vi "INIT_HP_2.vi"(4 "Averaging Number (8:256)":u32(ring) items=["1", "2", "4", "8", "16", "32", "64", "128", "256"], 6 "Integration Time":u32(ring)=2 items=["Short", "Medium", "Long"], 7 "Osc_Level [V]":dbl=0.02, 8 "Sweep Mode (0:Repeat)":u32(ring)=2 items=["Repeat", "Single", "Manual Point Mode"], 9 "Set":u32(ring)=7 caption="Selection A-B:" items=["| Z | -Ttheta ", "R - X", "Ls-Rs", "Ls-Q", "Cs-Rs", "Cs-Q", "Cs-D", "|Y|-Theta", "G-B", "Lp-G", "Lp-Q", "Cp-G", "Cp-Q", "Cp-D", "|Z|-Ls", "|Z|-Cs", "|Z|-Lp", "|Z|-Cp", "Lp-Rp", "Cp-Rp"], 10 "Reset Device (T:Reset Device)":bool, 11 "Type":u32(ring) caption="Measurement type" items=["Impedance ", "Gain - Phase", "Impedance With Probe"]) -> (0 "error out":errorcluster, 3 "VISA Refnum out":refnum<visa-resource-name>)   [LabVIEW 2017]
uses:
  ES2M_Auxetico/Lanzi_Romano/VI/Agilent 4194/Agilent 4194.lvlib
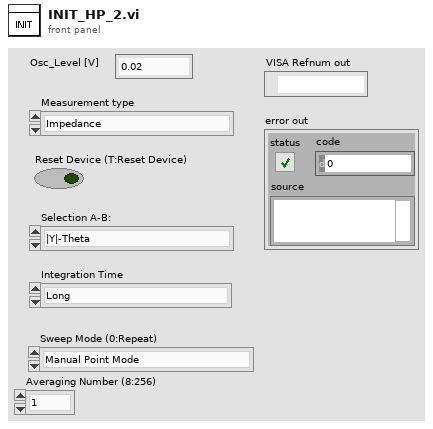
[diagram p1: front panel]
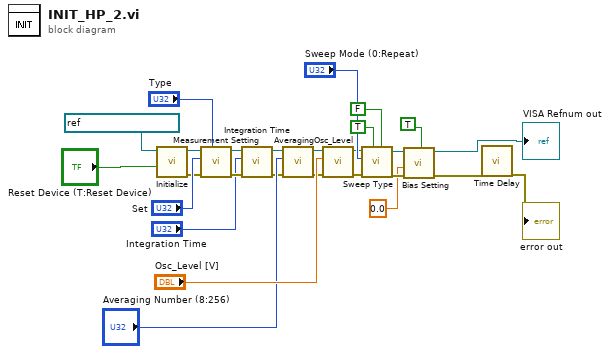
[diagram p0: block diagram]
diagram:
  n1 = call "Initialize.vi"("Reset Device (T:Reset Device)"="Reset Device (T:Reset Device)", "VISA resource name"=refnum<visa-resource-name> "GPIB0::17::INSTR") -> ("error out"=w5:errorcluster, "VISA resource name out"=w4:refnum<visa-resource-name>)  [unwired: 8 in]
  n2 = call "Measurement Setting.vi"("Measurement Type (0:Impedance)"="Type", "error in (no error)"=w5, "Impedance (0:| Z | - Theta )"="Set", "VISA resource name"=w4) -> ("error out"=w27:errorcluster, "VISA resource name out"=w26:refnum<visa-resource-name>)  [unwired: 6 in]
  n3 = call "Integration Time.vi"("error in (no error)"=w27, "Integration Time (0:Short)"="Integration Time", "VISA resource name"=w26) -> ("error out"=w8:errorcluster, "VISA resource name out"=w7:refnum<visa-resource-name>)  [unwired: 7 in]
  n4 = call "Averaging.vi"("error in (no error)"=w8, "Averaging Number (8:256)"="Averaging Number (8:256)", "VISA resource name"=w7) -> ("error out"=w11:errorcluster, "VISA resource name out"=w10:refnum<visa-resource-name>)  [unwired: 7 in]
  n5 = call "Osc_Level.vi"("error in (no error)"=w11, "Osc_Level [V]"="Osc_Level [V]", "VISA resource name"=w10) -> ("error out"=w15:errorcluster, "VISA resource name out"=w14:refnum<visa-resource-name>)  [unwired: 7 in]
  n6 = call "Sweep Type.vi"("Sweep Type (F:Linear)"=FALSE, "Sweep Direction (F:Down)"=TRUE, "error in (no error)"=w15, "Sweep Mode (0:Repeat)"="Sweep Mode (0:Repeat)", "VISA resource name"=w14) -> ("error out"=w21:errorcluster, "VISA resource name out"=w20:refnum<visa-resource-name>)  [unwired: 5 in]
  n7 = call "Bias Setting.vi"("error in (no error)"=w21, "DC Bias Value (0.0 V)"=0.0 ("BIAS [V]"), "DC Bias (F:Off)"=TRUE, "VISA resource name"=w20) -> ("error out"=w1:errorcluster, "VISA resource name out"=→"VISA Refnum out":refnum<visa-resource-name>)  [unwired: 6 in]
  n8 = call "Time Delay"("error in (no error)"=w1) -> ("error out"=→"error out":errorcluster)  [unwired: 10 in]
